vi "Logger Programatic Error Entry.vi"(11 "error in (no error)":errorcluster) -> (15 "error out":errorcluster)   [LabVIEW 2018]
uses:
  Log File Input.ctl
  Logger Global.vi
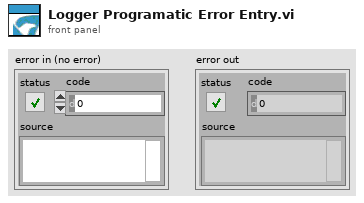
[diagram p1: front panel]
types:
  T1 = typedef "Log File Input.ctl" = cluster{"Log File Input":string, "Log Entry Type":enum16{"STANDARD", "WARNING", "CRITICAL"}}
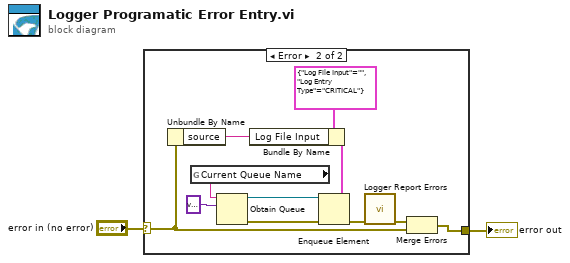
[diagram p0: block diagram]
diagram:
  n1 = case shown="Error" "error in (no error)" {
    selector: "error in (no error)" -> [w3 w9]
    tunnel: [w3 w10] -> w1
    frame No Error {
    }
    frame Error {
      n2 = Unbundle By Name(w9) -> ("source"=w6:string)
      n3 = global read "Logger Global.vi" "Current Queue Name"() -> (w12:string)
      n4 = Obtain Queue(name (unnamed)=w12, element data type=variant) -> (queue out=w13:refnum<queue>, error out=w14:errorcluster)  [unwired: 3 in, 1 out]
      n5 = Bundle By Name(cluster=T1 {"Log File Input"="", "Log Entry Type"=enum."CRITICAL"} ("Log File Input"), "Log File Input"=w6) -> (w8:T1)
      n6 = Enqueue Element(queue=w13, element=w8, error in (no error)=w14) -> (error out=w5:errorcluster)  [unwired: 1 in, 2 out]
      n7 = call "Logger Report Errors.vi"("error in (no error)"=w5) -> ("error out"=w4:errorcluster)  [unwired: 14 in]
      n8 = Merge Errors(w4, w9) -> (w10:errorcluster)
    }
  }
  "error out" <- w1
